vi "testDummy.vi"() -> ()   [LabVIEW 2020]
panel:
  out "Numeric":i32
  in  "stop":bool
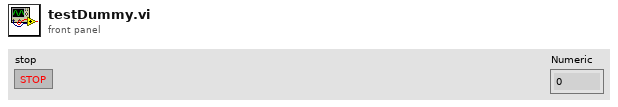
[diagram p1: front panel]
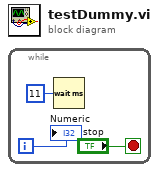
[diagram p0: block diagram]
diagram:
  n1 = while {
    i -> [w2]
    stop <- "stop" stop-if-true
    n2 = Wait (ms)(milliseconds to wait=u32 11) -> ()  [unwired: 1 out]
    "Numeric" <- w2
  }
